vi "Elevator Manual Command.vi"(7 "Description":string, 8 "Command Info In":T1, 9 "Deadband Value":dbl=0.01, 11 "Setpoint":dbl) -> (0 "Command Info Out":T1)   [LabVIEW 2018]
doc: "This template has a parameter to control whether it waits for the command to complete or not. This is useful for operations that have a timed duration or a sensor-based duration. \n\nBe sure to right-click and select New from Template and save with a new command name."
uses:
  <vilib>/Rock Robotics/WPI/Framework/Command Status Info.ctl
  <vilib>/Rock Robotics/WPI/Framework/Completion Status.ctl
  <vilib>/Rock Robotics/WPI/Framework/Completion Notifier.ctl
  Implementation/Subsystem Sequencer Setpoints.ctl
  Implementation/Subsystem Sequencer Operations.ctl
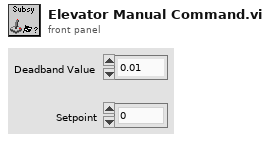
[diagram p1: front panel]
types:
  T1 = typedef "Command Status Info.ctl" = cluster{"Name":string, "Status":T2, "notifier out":T3}
  T2 = typedef "Completion Status.ctl" = enum16{"Successful", "Aborted", "Incomplete"}
  T3 = typedef "Completion Notifier.ctl" = refnum<notifier>
  T4 = typedef "Subsystem Sequencer Setpoints.ctl" = cluster{"Operation":T5, "Setpoint":dbl, "Duration":dbl}
  T5 = typedef "Subsystem Sequencer Operations.ctl" = enum16{"Reserve", "Read Current", "Run Sequence"}
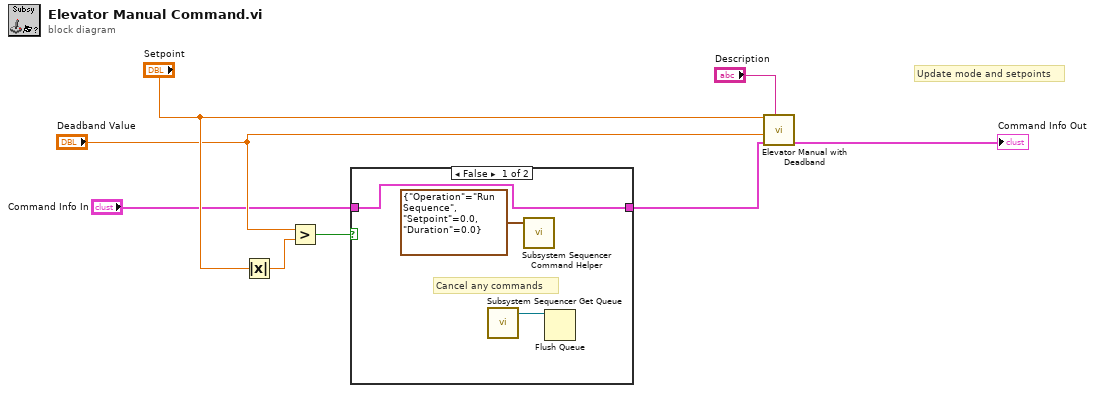
[diagram p0: block diagram]
diagram:
  # "Update mode and setpoints"
  n1 = Absolute Value(x="Setpoint") -> (abs(x)=w6:dbl)
  n2 = Greater?(x="Deadband Value", y=w6) -> (0:w3:bool)
  n3 = case shown="False" w3 {
    tunnel: "Command Info In" -> [w9 w12]
    tunnel: [w9 w12] -> w1
    frame False {
      # "Cancel any commands"
      n4 = call "Subsystem Sequencer Get Queue.vi"() -> ("queue out"=w11:refnum<queue>)  [unwired: 10 in, 1 out]
      n5 = call "Subsystem Sequencer Command Helper.vi"("SubSystem Data"=T4 {"Operation"=enum."Run Sequence", "Setpoint"=0.0, "Duration"=0.0}) -> ()  [unwired: 8 in, 3 out]
      n6 = Flush Queue(queue=w11) -> ()  [unwired: 1 in, 3 out]
    }
    frame True {
    }
  }
  n7 = call "Elevator Manual with Deadband.vi"("Description"="Description", "Command Info In"=w1, "Deadband Value"="Deadband Value", "Setpoint"="Setpoint") -> ("Command Info Out"=→"Command Info Out":T1)  [unwired: 7 in]
